vi "Get Table Range.vi"(7 "Sheet Name":string, 8 "error in":errorcluster, 10 "Table Identifier":string, 11 "SpreadsheetDoc in":refnum<k24>) -> (0 "error out":errorcluster, 2 "Range":string, 3 "SpreadsheetDoc out":refnum<k24>, 5 "Sheet Name":string)   [LabVIEW 2019, in "Open Xml.lvlib"]
uses:
  Open Xml.lvlib
  D:/git/Open-Xml-LabVIEW/Source/DocumentFormat.OpenXml.dll
  DocumentFormat.OpenXml.dll
  D:/git/Open-Xml-LabVIEW/Source/DocumentFormat.OpenXml.Framework.dll
  DocumentFormat.OpenXml.Framework.dll
panel:
  out "Value":u32
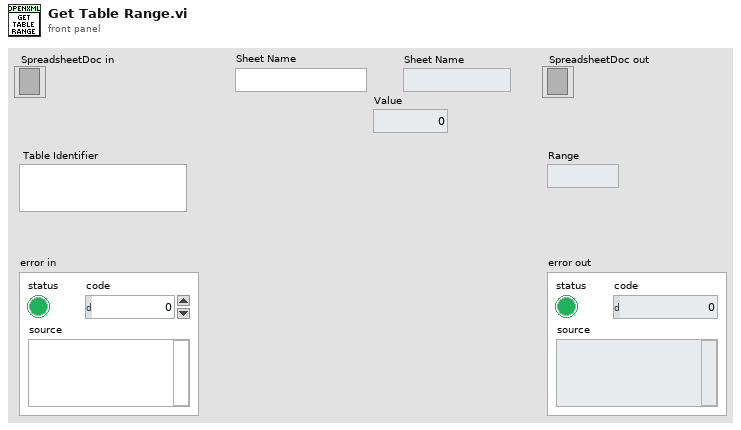
[diagram p1: front panel]
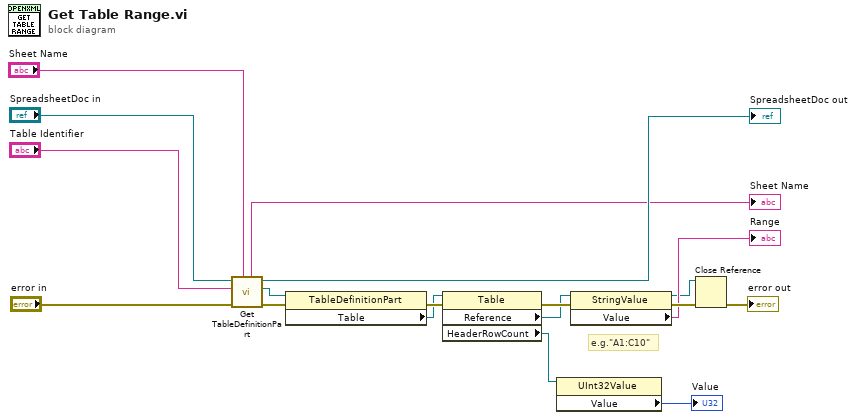
[diagram p0: block diagram]
diagram:
  # "e.g.\"A1:C10\""
  n1 = call "Get TableDefinitionPart.vi"("Sheet Name"="Sheet Name", "error in"="error in", "Table Name"="Table Identifier", "SpreadsheetDocument in"="SpreadsheetDoc in") -> ("error out"=w10:errorcluster, "TableDefinitionPart"=w8:refnum<k24>, "SpreadsheetDocument out"=→"SpreadsheetDoc out":refnum<k24>, "Sheet Name"=→"Sheet Name":string)  [unwired: 4 in]
  n2 = property class="TableDefinitionPart"(reference=w8, error in=w10) -> (error out=w9:errorcluster, "Table"=w6:refnum<k24>)  [unwired: 1 out]
  n3 = property class="Table"(reference=w6, error in=w9) -> (error out=w7:errorcluster, "Reference"=w5:refnum<k24>, "HeaderRowCount"=w2:refnum<k24>)  [unwired: 1 out]
  n4 = property class="UInt32Value"(reference=w2) -> ("Value"=→"Value":u32)  [unwired: 1 in, 2 out]
  n5 = property class="StringValue"(reference=w5, error in=w7) -> (reference out=w4:refnum<k24>, error out=w18:errorcluster, "Value"=→"Range":string)
  n6 = Close Reference(reference=w4, error in (no error)=w18) -> (error out=→"error out":errorcluster)
